vi "spectrometerTesting.vi"() -> ()   [LabVIEW 2020]
uses:
  <vilib>/Utility/file.llb/Write Delimited Spreadsheet (DBL).vi
  <instrlib>/Ocean Optics 2000 4000/Ocean Optics 2000 4000.lvlib
panel:
  in  "Enable Strobe (Disabled)":bool
  out "Spectral Waveform":cluster{dbl[], dbl[]}(graph)
  in  "VISA resource name":refnum<visa-resource-name>
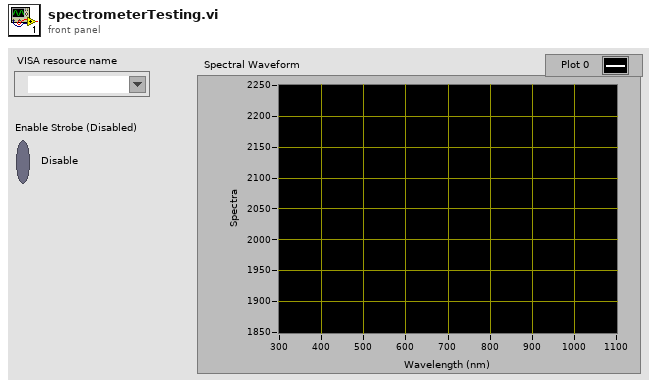
[diagram p1: front panel]
types:
  T1 = cluster{"Wavelength (nm)":dbl[], "Spectrum by Pixel Number":dbl[]}
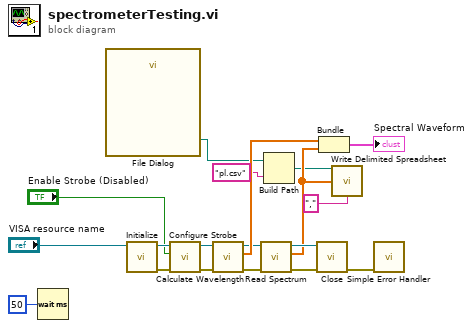
[diagram p0: block diagram]
diagram:
  n1 = Wait (ms)(milliseconds to wait=u32 50 ("millisecond multiple")) -> ()  [unwired: 1 out]
  n2 = call "File Dialog"() -> ("selected path"=w4:path)  [unwired: 12 in, 3 out]
  n3 = call <instrlib>:"Initialize.vi"("VISA resource name"="VISA resource name") -> ("error out"=w18:errorcluster, "VISA resource name out"=w19:refnum<visa-resource-name>)  [unwired: 2 in, 7 out]
  n4 = call <instrlib>:"Configure Strobe.vi"("error in (no error)"=w18, "Enable Strobe (Disabled)"="Enable Strobe (Disabled)", "VISA resource name"=w19) -> ("error out"=w8:errorcluster, "VISA resource name out"=w9:refnum<visa-resource-name>)  [unwired: 7 out]
  n5 = call <instrlib>:"Calculate Wavelength.vi"("error in (no error)"=w8, "VISA resource name"=w9) -> ("error out"=w10:errorcluster, "Wavelength (nm)"=w12:dbl[], "VISA resource name out"=w11:refnum<visa-resource-name>)  [unwired: 1 in, 6 out]
  n6 = call <instrlib>:"Read Spectrum.vi"("error in (no error)"=w10, "VISA resource name"=w11) -> ("error out"=w15:errorcluster, "Spectrum by Pixel Number"=w5:dbl[], "VISA resource name out"=w16:refnum<visa-resource-name>)  [unwired: 6 in, 1 out]
  n7 = Build Path(base path=w4, name or relative path="pl.csv") -> (appended path=w2:path)
  n8 = call <instrlib>:"Close.vi"("error in (no error)"=w15, "VISA resource name"=w16) -> ("error out"=w14:errorcluster)  [unwired: 9 out]
  n9 = Bundle("Wavelength (nm)"=w12, "Spectrum by Pixel Number"=w5) -> (→"Spectral Waveform":T1)  [unwired: 1 out]
  n10 = call-poly <vilib>:"Write Delimited Spreadsheet.vi"("file path (dialog if empty)"=w2, "1D data"=w5, "delimiter (\\t)"=",") -> ()  [unwired: 11 in, 2 out]
  n11 = call <vilib>:"Simple Error Handler.vi"("error in (no error)"=w14) -> ()  [unwired: 1 in, 8 out]
